vi "NET_Auto_Route.vi"(8 "Read(F) Write(T)":bool, 11 "Route In":T1) -> (3 "Route Out":T1)   [LabVIEW 2017]
uses:
  RoboRio Code/Systems/Autonomous/Autonomous/ENUM_Auto_AutoMode.ctl
  <vilib>/Rock Robotics/Network Tables/NT Read Number.vi
  <vilib>/Rock Robotics/Network Tables/NT Write Number.vi
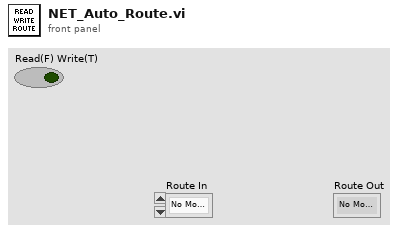
[diagram p1: front panel]
types:
  T1 = typedef "ENUM_Auto_AutoMode.ctl" = enum16{"No Movement", "Scale And Switch", "Switch", "Scale", "Cross Line"}
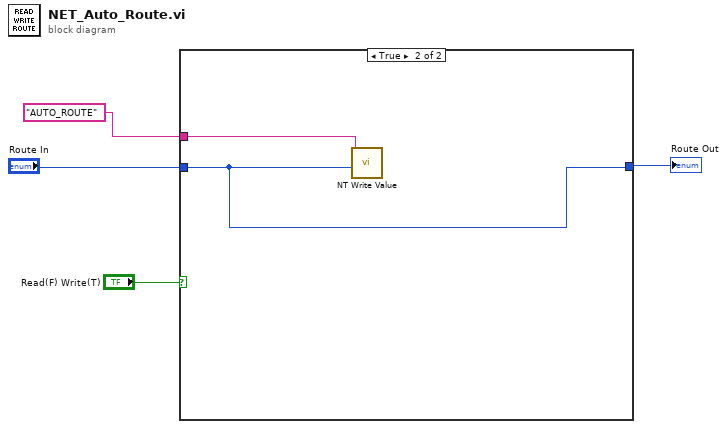
[diagram p0: block diagram]
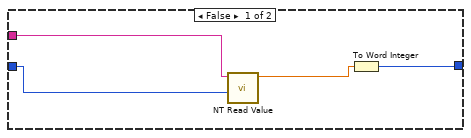
[diagram p2: hidden frame]
diagram:
  n1 = case shown="True" "Read(F) Write(T)" {
    tunnel: "AUTO_ROUTE" ("Name") -> [w8 w10]
    tunnel: "Route In" -> [w7 w9]
    tunnel: [w5 w9] -> w2
    frame False {
      n2 = call-poly <vilib>:"NT Read Value.vi"("Default Value"=w7, "Name"=w8) -> ("Numeric"=w6:dbl)  [unwired: 8 in, 1 out]
      n3 = To Word Integer(number=w6) -> (16bit integer=w5:i16)
    }
    frame True {
      n4 = call-poly <vilib>:"NT Write Value.vi"("Numeric"=w9, "Name"=w10) -> ()  [unwired: 9 in, 1 out]
    }
  }
  "Route Out" <- w2
